vi "http patch.vi"(0 "url":string, 1 "timeout_ms":i32, 5 "headers_json":string, 7 "body_ptr":string, 9 "body_len":i32, 11 "error in (no error)":errorcluster) -> (4 "response_len_out out":i32, 6 "status_out out":u32, 8 "function return":i32, 14 "handle_out out":u64, 15 "error out":errorcluster)   [LabVIEW 2020, in "reqwest-labview.lvlib"]
doc: "int http_patch(const char *url,\n const char *headers_json,\n const unsigned char *body_ptr,\n int body_len,\n int timeout_ms,\n void **handle_out,\n int *response_len_out,\n unsigned int *status_out);"
uses:
  reqwest-labview.lvlib
  lib_reqwest_labview_64.dll
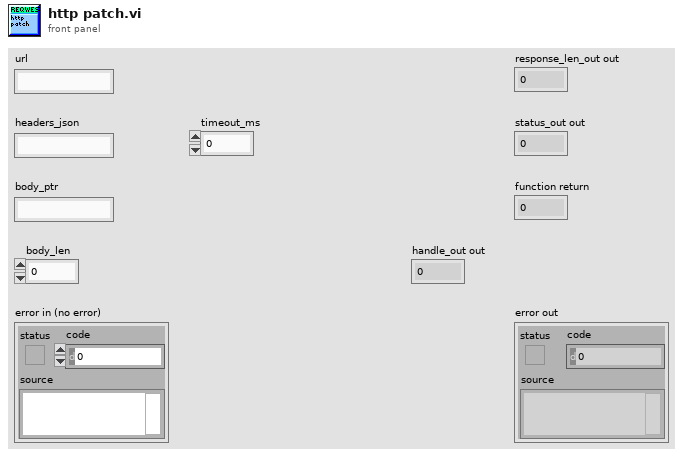
[diagram p1: front panel]
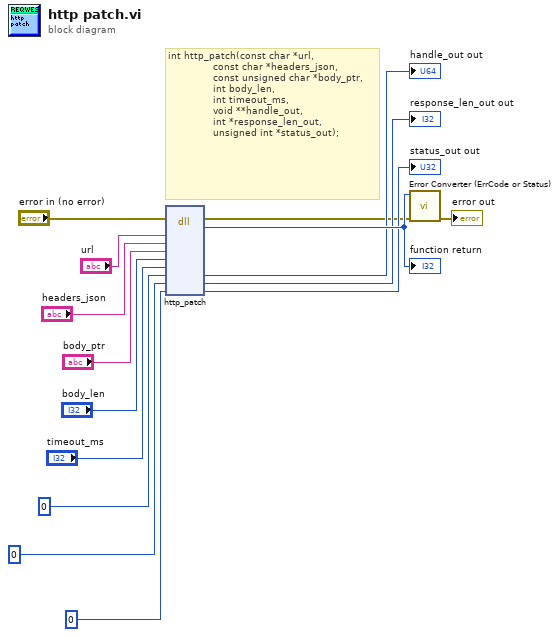
[diagram p0: block diagram]
diagram:
  # "int http_patch(const char *url,\n               const char *headers_json,\n               const unsigned char *body_ptr,\n               int body_len,\n               int timeout_ms,\n               void **handle_out,\n               int *response_len_out,\n               unsigned int *status_out);"
  n1 = dll-call lib="C:/code/reqwest-labview/lv-src/shared-library/lib_reqwest_labview_*.*" fn="http_patch"(error in="error in (no error)", "url"="url", "headers_json"="headers_json", "body_ptr"="body_ptr", "body_len"="body_len", "timeout_ms"="timeout_ms", "handle_out"=u64 0, "response_len_out"=0, "status_out"=u32 0) -> (error out=w2:errorcluster, "return type"=w15:i32, "handle_out"=→"handle_out out":u64, "response_len_out"=→"response_len_out out":i32, "status_out"=→"status_out out":u32)  [unwired: 7 in, 1 out]
  "function return" <- w15
  n2 = call "Error Converter (ErrCode or Status).vi"("error in (no error)"=w2, "error code"=w15) -> ("error out"=→"error out":errorcluster)  [unwired: 9 in]
